vi "VC Elapsed Time.vi"(11 "AM Refs in":T1) -> (1 "Time has Elapsed":bool, 3 "AM Refs in":T1, 4 "Elapsed Time (s)":dbl)   [LabVIEW 2020, in "Valve Control.lvlib"]
uses:
  Valve Control.lvlib
  AM Configuration.ctl
  support/Message Queue/Message Cluster.ctl
  support/Message Queue/Message Queue.lvlib
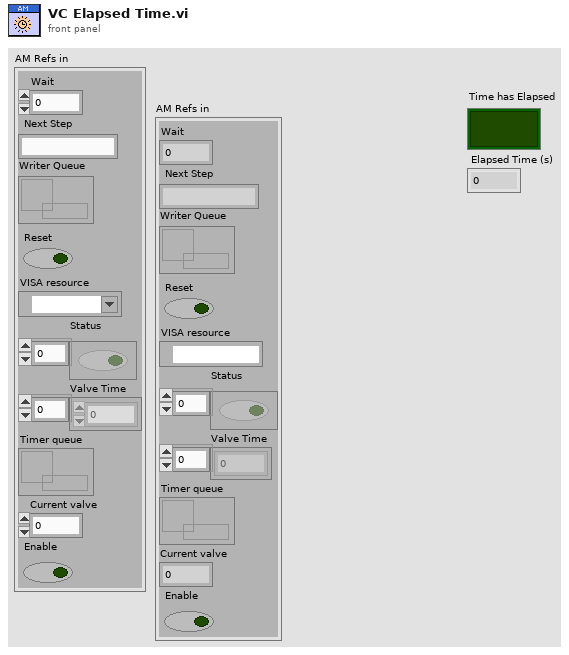
[diagram p1: front panel]
types:
  T1 = typedef "Valve Control.lvlib/AM Configuration.ctl" = cluster{"Wait":dbl, "Next Step":string, "Writer Queue":refnum<queue>, "Reset":bool, "VISA resource":refnum<visa-resource-name>, "Status":bool[], "Valve Time":dbl[], "Timer queue":refnum<queue>, "Current valve":i32, "Enable":bool}
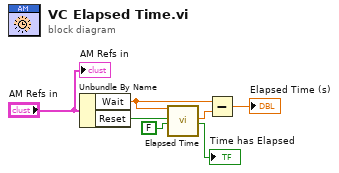
[diagram p0: block diagram]
diagram:
  n1 = Unbundle By Name("AM Refs in") -> ("Wait"=w1:dbl, "Reset"=w5:bool)
  n2 = call "Elapsed Time"("Time Target (s)"=w1, "Reset"=w5, "Auto Reset"=FALSE) -> ("Elapsed Time (s)"=w3:dbl, "Time has Elapsed"=→"Time has Elapsed":bool)  [unwired: 9 in, 6 out]
  n3 = Subtract(x=w1, y=w3) -> (x-y=→"Elapsed Time (s)":dbl)
  "AM Refs in" <- "AM Refs in"
